vi "Max Lines.vi"(8 "scan mode in":i32=-1, 9 "Camera Model":string="C14440-20UP", 10 "Frame Time (ms)":dbl=100.0 min=0.06822 max=10000.0, 11 "Duty cycle (fraction)":dbl=1.0 min=0.06822 max=10000.0) -> (0 "scan mode out":i32, 1 "upper limit":i32=2048, 2 "Max Lines":i32=168, 3 "Exposure Time (ms)":dbl=0.0682105 min=0.06822 max=10000.0, 4 "Allowed scan modes":cluster{"String":string, "Number":i32}[](array[cluster]), 5 "unbinned image width":i32)   [LabVIEW 2018]
panel:
  out "Allowed Scan Modes":u16(ring) items=["Auto"=65535, "Slow"=1, "Standard"=2]
  out "Target frame readout time (ms)":dbl
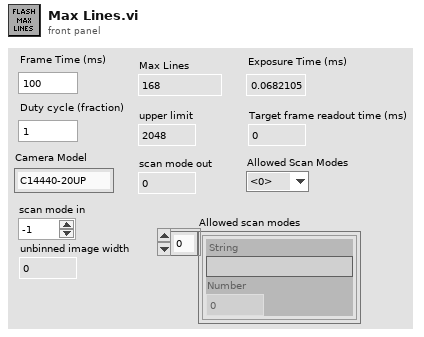
[diagram p1: front panel]
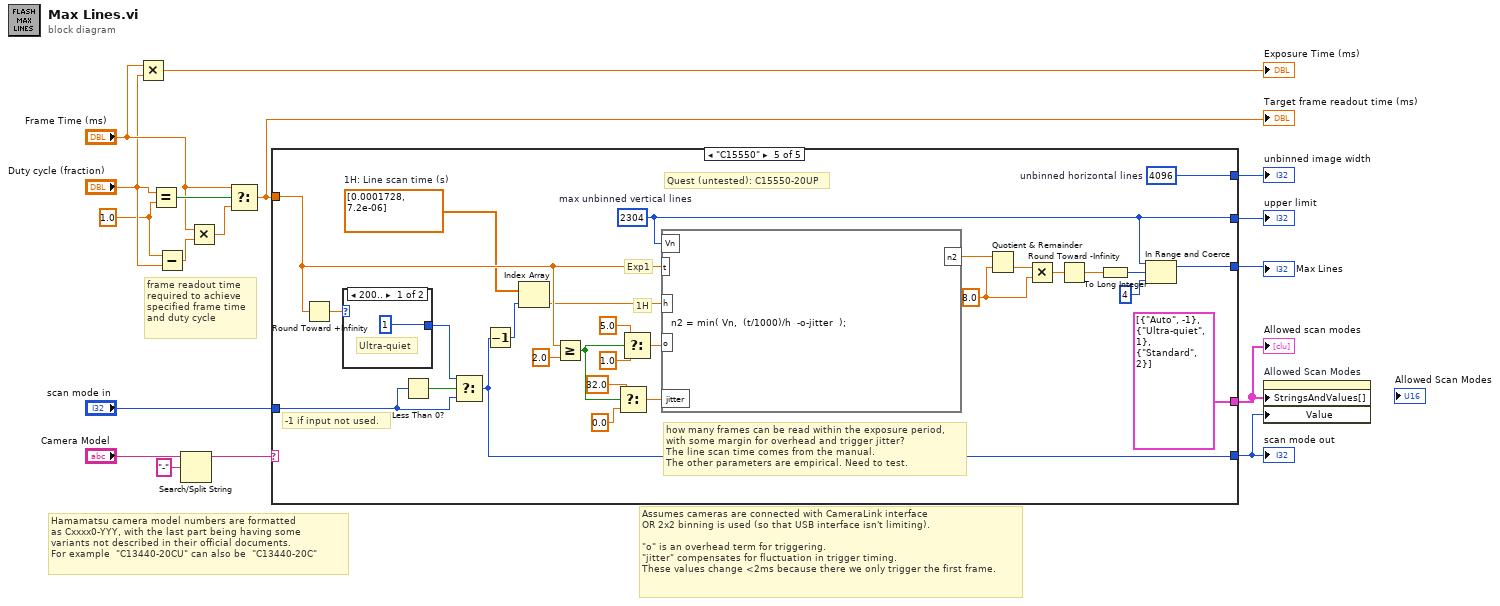
[diagram p0: block diagram]
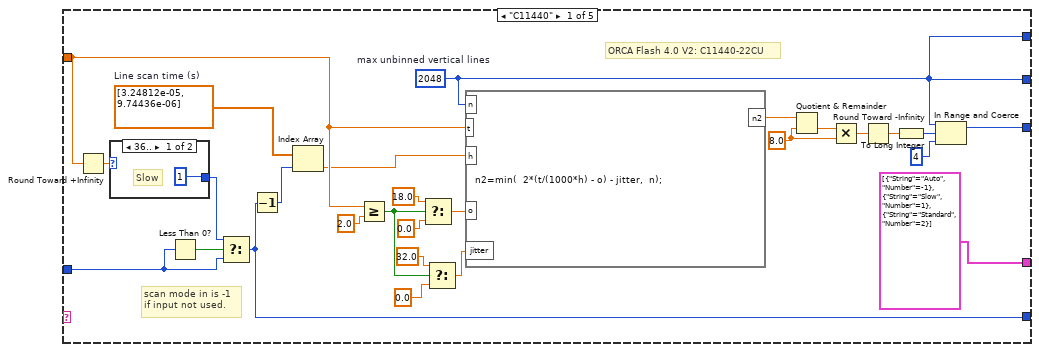
[diagram p2: hidden frame]
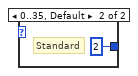
[diagram p3: hidden frame]
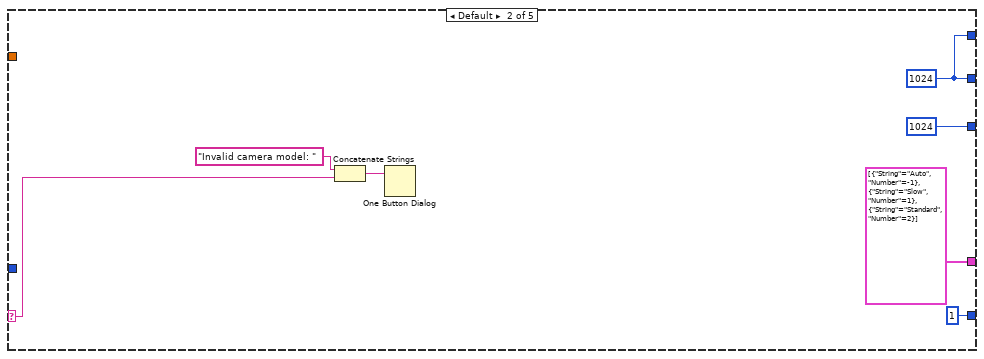
[diagram p4: hidden frame]
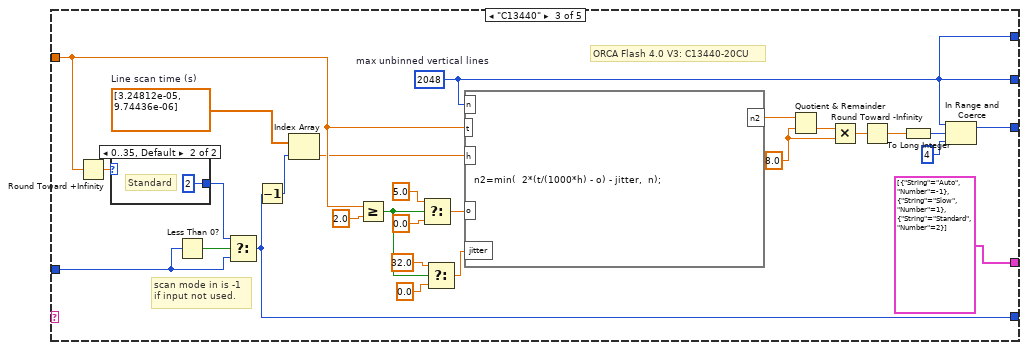
[diagram p5: hidden frame]
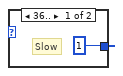
[diagram p6: hidden frame]
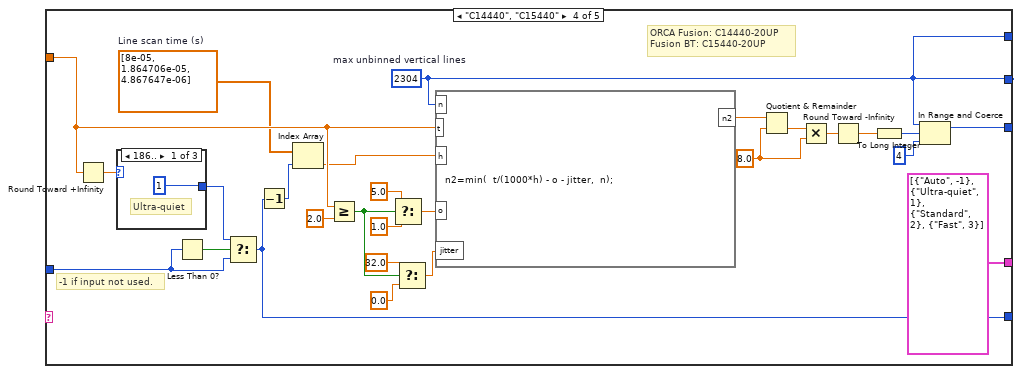
[diagram p7: hidden frame]
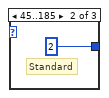
[diagram p8: hidden frame]
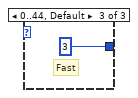
[diagram p9: hidden frame]
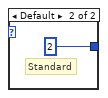
[diagram p10: hidden frame]
diagram:
  w8 = 1.0 ("y")
  # "Hamamatsu camera model numbers are formatted\nas Cxxxx0-YYY, with the last part being having some\nvariants not described in their official documents.\nFor example  \"C13440-20CU\" can also be  \"C13440-20C\""
  # "frame readout time\nrequired to achieve\nspecified frame time\nand duty cycle"
  # "Assumes cameras are connected with CameraLink interface\nOR 2x2 binning is used (so that USB interface isn't limiting).\n\n\"o\" is an overhead term for triggering.\n\"jitter\" compensates for fluctuation in trigger timing.\nThese values change <2ms because there we only trigger the first frame."
  n1 = Multiply(x="Frame Time (ms)", y="Duty cycle (fraction)") -> (x*y=→"Exposure Time (ms)":dbl)
  n2 = Equal?(x="Duty cycle (fraction)", y=w8) -> (x = y?=w15:bool)
  n3 = Subtract(x=w8, y="Duty cycle (fraction)") -> (x-y=w12:dbl)
  n4 = Search/Split String(string="Camera Model", search string/char (-)="-") -> (substring before match=w3:string)  [unwired: 1 in, 2 out]
  n5 = Multiply(x="Frame Time (ms)", y=w12) -> (x*y=w10:dbl)
  n6 = Select(t="Frame Time (ms)", s=w15, f=w10) -> (s? t:f=w14:dbl)
  "Target frame readout time (ms)" <- w14
  n7 = case shown="\"C15550\"" w3 {
    selector: w3 -> [_ w50 _ _ _]
    tunnel: w14 -> [w26 _ w62 w93 w130]
    tunnel: [w31 1024 ("max unbinned vertical lines") w66 w96 w132] -> w17
    tunnel: [w18 w47 w54 w83 w131] -> w16
    tunnel: [w20 1 ("scan mode in") w58 w85 w121] -> w5
    tunnel: "scan mode in" -> [w23 _ w61 w89 w126]
    tunnel: [cluster{"String":string, "Number":i32}[] [{"String"="Auto", "Number"=-1}, {"String"="Slow", "Number"=1}, {"String"="Standard", "Number"=2}] cluster{"String":string, "Number":i32}[] [{"String"="Auto", "Number"=-1}, {"String"="Slow", "Number"=1}, {"String"="Standard", "Number"=2}] cluster{"String":string, "Number":i32}[] [{"String"="Auto", "Number"=-1}, {"String"="Slow", "Number"=1}, {"String"="Standard", "Number"=2}] cluster{"String":string, "Number":i32}[] [{"String"="Auto", "Number"=-1}, {"String"="Ultra-quiet", "Number"=1}, {"String"="Standard", "Number"=2}, {"String"="Fast", "Number"=3}] cluster{"String":string, "Number":i32}[] [{"String"="Auto", "Number"=-1}, {"String"="Ultra-quiet", "Number"=1}, {"String"="Standard", "Number"=2}]] -> w7
    tunnel: [w18 w47 w54 w83 w113] -> w1
    frame "C11440" {
      w25 = dbl[] [3.24812e-05, 9.74436e-06]  # Line scan time (s)
      w18 = 2048  # max unbinned vertical lines
      w43 = 8.0 ("y")
      # "scan mode in is -1\nif input not used."
      # "ORCA Flash 4.0 V2: C11440-22CU"
      n8 = Round Toward +Infinity(x=w26) -> (ceil(x): smallest int >= x=w27:dbl)
      n9 = case shown="36.." w27 {
        tunnel: [1 ("lower limit") 2 ("lower limit")] -> w28
        frame 36.. {
          # "Slow"
        }
        frame 0..35, Default {
          # "Standard"
        }
      }
      n10 = Less Than 0?(x=w23) -> (x < 0?=w29:bool)
      n11 = Select(t=w28, s=w29, f=w23) -> (s? t:f=w20:i32)
      n12 = Decrement(x=w20) -> (x-1=w21:i32)
      n13 = Index Array(array=w25, index=w21) -> (element=w24:dbl)
      n14 = Greater Or Equal?(x=w26, y=2.0) -> (x >= y?=w36:bool)
      n15 = Select(t=18.0 ("f"), s=w36, f=0.0) -> (s? t:f=w34:dbl)
      n16 = Select(t=32.0 ("input variable"), s=w36, f=0.0) -> (s? t:f=w35:dbl)
      n17 = formula code="n2=min(  2*(t/(1000*h) - o) - jitter,  n);"("t"=w26, "h"=w24, "n"=w18, "o"=w34, "jitter"=w35) -> ("n2"=w42:dbl)
      n18 = Quotient & Remainder(x=w42, y=w43) -> (floor(x/y)=w44:dbl)  [unwired: 1 out]
      n19 = Multiply(x=w44, y=w43) -> (x*y=w41:dbl)
      n20 = Round Toward -Infinity(1:w41) -> (0:w40:dbl)
      n21 = To Long Integer(number=w40) -> (32bit integer=w32:i32)
      n22 = In Range and Coerce(upper limit=w18, x=w32, lower limit=4) -> (coerced(x)=w31:i32)  [unwired: 1 out]
    }
    frame Default {
      w47 = 1024 ("max unbinned vertical lines")
      n23 = Concatenate Strings("Invalid camera model: " ("message"), w50) -> (w48:string)
      n24 = One Button Dialog(message=w48) -> ()  [unwired: 1 in, 1 out]
    }
    frame "C13440" {
      w63 = dbl[] [3.24812e-05, 9.74436e-06]  # Line scan time (s)
      w54 = 2048  # max unbinned vertical lines
      w79 = 8.0 ("y")
      # "scan mode in is -1\nif input not used."
      # "ORCA Flash 4.0 V3: C13440-20CU"
      n25 = Round Toward +Infinity(x=w62) -> (ceil(x): smallest int >= x=w56:dbl)
      n26 = case shown="0..35, Default" w56 {
        tunnel: [1 ("lower limit") 2 ("lower limit")] -> w55
        frame 36.. {
          # "Slow"
        }
        frame 0..35, Default {
          # "Standard"
        }
      }
      n27 = Less Than 0?(x=w61) -> (x < 0?=w64:bool)
      n28 = Select(t=w55, s=w64, f=w61) -> (s? t:f=w58:i32)
      n29 = Decrement(x=w58) -> (x-1=w59:i32)
      n30 = Index Array(array=w63, index=w59) -> (element=w60:dbl)
      n31 = Greater Or Equal?(x=w62, y=2.0) -> (x >= y?=w72:bool)
      n32 = Select(t=5.0 ("f"), s=w72, f=0.0) -> (s? t:f=w70:dbl)
      n33 = Select(t=32.0 ("input variable"), s=w72, f=0.0) -> (s? t:f=w71:dbl)
      n34 = formula code="n2=min(  2*(t/(1000*h) - o) - jitter,  n);"("t"=w62, "h"=w60, "n"=w54, "o"=w70, "jitter"=w71) -> ("n2"=w78:dbl)
      n35 = Quotient & Remainder(x=w78, y=w79) -> (floor(x/y)=w80:dbl)  [unwired: 1 out]
      n36 = Multiply(x=w80, y=w79) -> (x*y=w77:dbl)
      n37 = Round Toward -Infinity(1:w77) -> (0:w76:dbl)
      n38 = To Long Integer(number=w76) -> (32bit integer=w68:i32)
      n39 = In Range and Coerce(upper limit=w54, x=w68, lower limit=4) -> (coerced(x)=w66:i32)  [unwired: 1 out]
    }
    frame "C14440", "C15440" {
      w88 = dbl[] [8e-05, 1.864706e-05, 4.867647e-06]  # Line scan time (s)
      w83 = 2304  # max unbinned vertical lines
      w103 = 8.0 ("y")
      # "-1 if input not used."
      # "ORCA Fusion: C14440-20UP\nFusion BT: C15440-20UP"
      n40 = Round Toward +Infinity(x=w93) -> (ceil(x): smallest int >= x=w92:dbl)
      n41 = case shown="186.." w92 {
        tunnel: [1 ("lower limit") 2 ("lower limit") 3 ("lower limit")] -> w91
        frame 186.. {
          # "Ultra-quiet"
        }
        frame 45..185 {
          # "Standard"
        }
        frame 0..44, Default {
          # "Fast"
        }
      }
      n42 = Less Than 0?(x=w89) -> (x < 0?=w90:bool)
      n43 = Select(t=w91, s=w90, f=w89) -> (s? t:f=w85:i32)
      n44 = Decrement(x=w85) -> (x-1=w86:i32)
      n45 = Index Array(array=w88, index=w86) -> (element=w87:dbl)
      n46 = Greater Or Equal?(x=w93, y=2.0) -> (x >= y?=w108:bool)
      n47 = Select(t=5.0 ("f"), s=w108, f=1.0) -> (s? t:f=w95:dbl)
      n48 = Select(t=32.0 ("input variable"), s=w108, f=0.0) -> (s? t:f=w94:dbl)
      n49 = formula code="n2=min(  t/(1000*h) - o - jitter,  n);"("t"=w93, "h"=w87, "n"=w83, "o"=w95, "jitter"=w94) -> ("n2"=w105:dbl)
      n50 = Quotient & Remainder(x=w105, y=w103) -> (floor(x/y)=w104:dbl)  [unwired: 1 out]
      n51 = Multiply(x=w104, y=w103) -> (x*y=w106:dbl)
      n52 = Round Toward -Infinity(1:w106) -> (0:w107:dbl)
      n53 = To Long Integer(number=w107) -> (32bit integer=w109:i32)
      n54 = In Range and Coerce(upper limit=w83, x=w109, lower limit=4) -> (coerced(x)=w96:i32)  [unwired: 1 out]
    }
    frame "C15550" {
      w113 = 4096  # unbinned horizontal lines
      w125 = dbl[] [0.0001728, 7.2e-06]  # 1H: Line scan time (s)
      w131 = 2304  # max unbinned vertical lines
      w135 = 8.0 ("y")
      # "how many frames can be read within the exposure period,\nwith some margin for overhead and trigger jitter?\nThe line scan time comes from the manual.\nThe other parameters are empirical. Need to test."
      # "1H"
      # "Exp1"
      # "-1 if input not used."
      # "Quest (untested): C15550-20UP"
      n55 = Round Toward +Infinity(x=w130) -> (ceil(x): smallest int >= x=w129:dbl)
      n56 = case shown="200.." w129 {
        tunnel: [1 ("lower limit") 2 ("lower limit")] -> w128
        frame 200.. {
          # "Ultra-quiet"
        }
        frame Default {
          # "Standard"
        }
      }
      n57 = Less Than 0?(x=w126) -> (x < 0?=w127:bool)
      n58 = Select(t=w128, s=w127, f=w126) -> (s? t:f=w121:i32)
      n59 = Decrement(x=w121) -> (x-1=w123:i32)
      n60 = Index Array(array=w125, index=w123) -> (element=w124:dbl)
      n61 = Greater Or Equal?(x=w130, y=2.0) -> (x >= y?=w114:bool)
      n62 = Select(t=32.0 ("input variable"), s=w114, f=0.0) -> (s? t:f=w118:dbl)
      n63 = Select(t=5.0 ("f"), s=w114, f=1.0) -> (s? t:f=w115:dbl)
      n64 = formula code="n2 = min( Vn,  (t/1000)/h  -o-jitter  );"("t"=w130, "h"=w124, "Vn"=w131, "jitter"=w118, "o"=w115) -> ("n2"=w137:dbl)
      n65 = Quotient & Remainder(x=w137, y=w135) -> (floor(x/y)=w136:dbl)  [unwired: 1 out]
      n66 = Multiply(x=w136, y=w135) -> (x*y=w138:dbl)
      n67 = Round Toward -Infinity(1:w138) -> (0:w139:dbl)
      n68 = To Long Integer(number=w139) -> (32bit integer=w140:i32)
      n69 = In Range and Coerce(upper limit=w131, x=w140, lower limit=4) -> (coerced(x)=w132:i32)  [unwired: 1 out]
    }
  }
  "Max Lines" <- w17
  "upper limit" <- w16
  "scan mode out" <- w5
  "Allowed scan modes" <- w7
  "unbinned image width" <- w1
  n70 = property on="Allowed Scan Modes" class="Ring (strict)"("StringsAndValues[]"=w7, "Value"=w5) -> ()  [unwired: 2 in, 2 out]
